vi "WaveformWriteToSpreedSheet.vi"() -> ()   [LabVIEW 2019]
uses:
  <vilib>/Waveform/WDTFileIO.llb/Export Waveform To Spreadsheet File.vi
  <vilib>/measure/NI_MABase.lvlib
panel:
  out "error out":errorcluster
  out "Waveform Graph":waveform(dbl)(graph)
  in  "file path (dialog if empty)":path
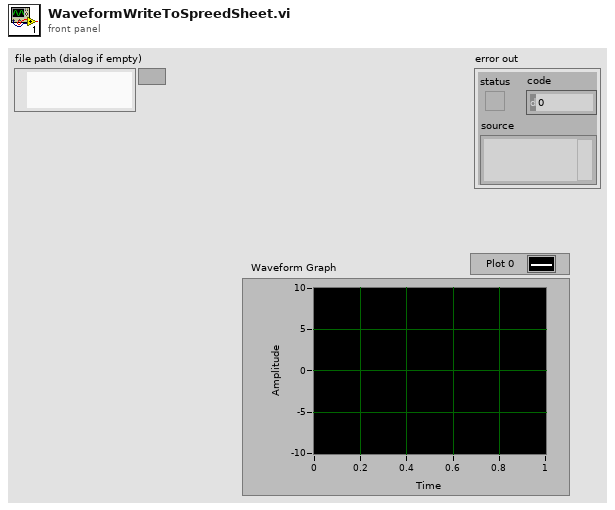
[diagram p1: front panel]
types:
  T1 = enum16{"Sine Wave", "Triangle Wave", "Square Wave", "Sawtooth Wave"}
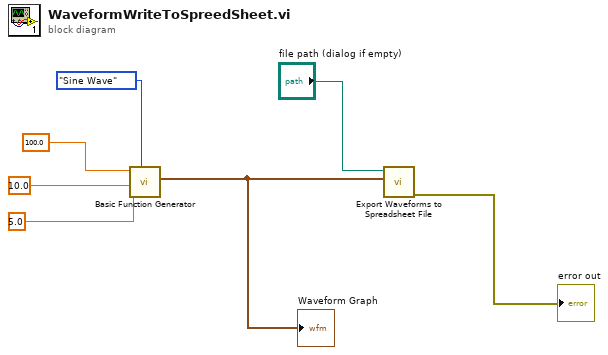
[diagram p0: block diagram]
diagram:
  n1 = call <vilib>:"Basic Function Generator.vi"("signal type"=T1."Sine Wave", "phase"=5.0, "amplitude"=10.0, "frequency"=100.0) -> ("signal out"=w2:waveform(dbl))  [unwired: 5 in, 2 out]
  "Waveform Graph" <- w2
  n2 = call-poly <vilib>:"Export Waveforms to Spreadsheet File.vi"("waveform"=w2, "file path (dialog if empty)"="file path (dialog if empty)") -> ("error out"=→"error out":errorcluster)  [unwired: 8 in, 1 out]
